vi "AuMT8852B EDR Rel Outp Pwr Extended Test.vi"() -> ()   [LabVIEW 2017]
doc: "This example shows how to extract Extended Test Results by using multiple 'Results Panels', each configurable via the 'Stage' Configuration Input control. Note that the 'Configuration Settings' (i.e. Use Low/Medium/High Frequency), must be enabled in order to obtain valid test results in the appropriate 'Test Results' output panel."
panel:
  out "error out":errorcluster
  in  "Settings":T1={"Low frequency selection"=enum."Use low frequency", "Medium frequency selection"=enum."Use medium frequency", "High frequency selection"=enum."Use high frequency", "Low TX frequency"=2402.0, "Low RX frequency"=2480.0, "Medium TX frequency"=2441.0, "Medium RX frequency"=2402.0, "High TX frequency"=2480.0, "High RX frequency"=2402.0, "Number of packets"=10, "PDPSK-PGFSK upper limit (dB) "=1.0, "PDPSK-PGFSK lower limit (dB)"=4.0, "2DHx test packet"=enum."Longest", "3DHx test packet"=enum."Longest", "Hop selection"=enum."Test with hopping off and on", "Test control"=enum."Loopback", "Hop mode"=enum."Defined", "Output Power Level"=enum."Max & Min"} {"PDPSK-PGFSK lower limit (dB)" format="%.2f"; "PDPSK-PGFSK upper limit (dB)" format="%.2f"}
  out "Addresses":string[](array[string])
  in  "Start/Stop (Start)":enum16{"Start", "Stop"}(ring)
  in  "Test Results":T2(tab)=enum."Hopon any Max"
  in  "Stage 1":T3(ring)
  out "Results 1":T4 {"Peak 2DHx DPSK Absolute Power (dBm)" format="%.2f"; "Avg 2DHx DPSK Absolute Power (dBm)" format="%.2f"; "Min 2DHx DPSK Absolute Power (dBm)" format="%.2f"; "Max 2DHx DPSK Absolute Power (dBm)" format="%.2f"; "Peak 2DHx GFSK Absolute Power (dBm)" format="%.2f"; "Avg 2DHx GFSK Absolute Power (dBm)" format="%.2f"; "Min 2DHx GFSK Absolute Power (dBm)" format="%.2f"; "Max 2DHx GFSK Absolute Power (dBm)" format="%.2f"; "Peak 3DHx DPSK Absolute Power (dBm)" format="%.2f"; "Avg 3DHx DPSK Absolute Power (dBm)" format="%.2f"; "Min 3DHx DPSK Absolute Power (dBm)" format="%.2f"; "Max 3DHx DPSK Absolute Power (dBm)" format="%.2f"; "Peak 3DHx GFSK Absolute Power (dBm)" format="%.2f"; "Avg 3DHx GFSK Absolute Power (dBm)" format="%.2f"; "Min 3DHx GFSK Absolute Power (dBm)" format="%.2f"; "Max 3DHx GFSK Absolute Power (dBm)" format="%.2f"; "Avg power difference (dBm)" format="%.2f"; "Min power difference (dBm)" format="%.2f"; "Max power difference (dBm)" format="%.2f"; "Avg power difference (dBm)" format="%.2f"; "Min power difference (dBm)" format="%.2f"; "Max power difference (dBm)" format="%.2f"}
  in  "Stage 2":T3(ring)=enum."Hop off defined low frequency EUT Max"
  out "Results  2":T4 {"Peak 2DHx DPSK Absolute Power (dBm)" format="%.2f"; "Avg 2DHx DPSK Absolute Power (dBm)" format="%.2f"; "Min 2DHx DPSK Absolute Power (dBm)" format="%.2f"; "Max 2DHx DPSK Absolute Power (dBm)" format="%.2f"; "Peak 2DHx GFSK Absolute Power (dBm)" format="%.2f"; "Avg 2DHx GFSK Absolute Power (dBm)" format="%.2f"; "Min 2DHx GFSK Absolute Power (dBm)" format="%.2f"; "Max 2DHx GFSK Absolute Power (dBm)" format="%.2f"; "Peak 3DHx DPSK Absolute Power (dBm)" format="%.2f"; "Avg 3DHx DPSK Absolute Power (dBm)" format="%.2f"; "Min 3DHx DPSK Absolute Power (dBm)" format="%.2f"; "Max 3DHx DPSK Absolute Power (dBm)" format="%.2f"; "Peak 3DHx GFSK Absolute Power (dBm)" format="%.2f"; "Avg 3DHx GFSK Absolute Power (dBm)" format="%.2f"; "Min 3DHx GFSK Absolute Power (dBm)" format="%.2f"; "Max 3DHx GFSK Absolute Power (dBm)" format="%.2f"; "Avg power difference (dBm)" format="%.2f"; "Min power difference (dBm)" format="%.2f"; "Max power difference (dBm)" format="%.2f"; "Avg power difference (dBm)" format="%.2f"; "Min power difference (dBm)" format="%.2f"; "Max power difference (dBm)" format="%.2f"}
  in  "Stage 3":T3(ring)=enum."Hop off defined medium frequency EUT Min"
  out "Results  3":T4 {"Peak 2DHx DPSK Absolute Power (dBm)" format="%.2f"; "Avg 2DHx DPSK Absolute Power (dBm)" format="%.2f"; "Min 2DHx DPSK Absolute Power (dBm)" format="%.2f"; "Max 2DHx DPSK Absolute Power (dBm)" format="%.2f"; "Peak 2DHx GFSK Absolute Power (dBm)" format="%.2f"; "Avg 2DHx GFSK Absolute Power (dBm)" format="%.2f"; "Min 2DHx GFSK Absolute Power (dBm)" format="%.2f"; "Max 2DHx GFSK Absolute Power (dBm)" format="%.2f"; "Peak 3DHx DPSK Absolute Power (dBm)" format="%.2f"; "Avg 3DHx DPSK Absolute Power (dBm)" format="%.2f"; "Min 3DHx DPSK Absolute Power (dBm)" format="%.2f"; "Max 3DHx DPSK Absolute Power (dBm)" format="%.2f"; "Peak 3DHx GFSK Absolute Power (dBm)" format="%.2f"; "Avg 3DHx GFSK Absolute Power (dBm)" format="%.2f"; "Min 3DHx GFSK Absolute Power (dBm)" format="%.2f"; "Max 3DHx GFSK Absolute Power (dBm)" format="%.2f"; "Avg power difference (dBm)" format="%.2f"; "Min power difference (dBm)" format="%.2f"; "Max power difference (dBm)" format="%.2f"; "Avg power difference (dBm)" format="%.2f"; "Min power difference (dBm)" format="%.2f"; "Max power difference (dBm)" format="%.2f"}
  in  "Stage 4":T3(ring)=enum."Hop off defined medium frequency EUT Max"
  out "Results  4":T4 {"Peak 2DHx DPSK Absolute Power (dBm)" format="%.2f"; "Avg 2DHx DPSK Absolute Power (dBm)" format="%.2f"; "Min 2DHx DPSK Absolute Power (dBm)" format="%.2f"; "Max 2DHx DPSK Absolute Power (dBm)" format="%.2f"; "Peak 2DHx GFSK Absolute Power (dBm)" format="%.2f"; "Avg 2DHx GFSK Absolute Power (dBm)" format="%.2f"; "Min 2DHx GFSK Absolute Power (dBm)" format="%.2f"; "Max 2DHx GFSK Absolute Power (dBm)" format="%.2f"; "Peak 3DHx DPSK Absolute Power (dBm)" format="%.2f"; "Avg 3DHx DPSK Absolute Power (dBm)" format="%.2f"; "Min 3DHx DPSK Absolute Power (dBm)" format="%.2f"; "Max 3DHx DPSK Absolute Power (dBm)" format="%.2f"; "Peak 3DHx GFSK Absolute Power (dBm)" format="%.2f"; "Avg 3DHx GFSK Absolute Power (dBm)" format="%.2f"; "Min 3DHx GFSK Absolute Power (dBm)" format="%.2f"; "Max 3DHx GFSK Absolute Power (dBm)" format="%.2f"; "Avg power difference (dBm)" format="%.2f"; "Min power difference (dBm)" format="%.2f"; "Max power difference (dBm)" format="%.2f"; "Avg power difference (dBm)" format="%.2f"; "Min power difference (dBm)" format="%.2f"; "Max power difference (dBm)" format="%.2f"}
  in  "Stage 5":T3(ring)=enum."Hop off defined high frequency EUT Min"
  out "Results  5":T4 {"Peak 2DHx DPSK Absolute Power (dBm)" format="%.2f"; "Avg 2DHx DPSK Absolute Power (dBm)" format="%.2f"; "Min 2DHx DPSK Absolute Power (dBm)" format="%.2f"; "Max 2DHx DPSK Absolute Power (dBm)" format="%.2f"; "Peak 2DHx GFSK Absolute Power (dBm)" format="%.2f"; "Avg 2DHx GFSK Absolute Power (dBm)" format="%.2f"; "Min 2DHx GFSK Absolute Power (dBm)" format="%.2f"; "Max 2DHx GFSK Absolute Power (dBm)" format="%.2f"; "Peak 3DHx DPSK Absolute Power (dBm)" format="%.2f"; "Avg 3DHx DPSK Absolute Power (dBm)" format="%.2f"; "Min 3DHx DPSK Absolute Power (dBm)" format="%.2f"; "Max 3DHx DPSK Absolute Power (dBm)" format="%.2f"; "Peak 3DHx GFSK Absolute Power (dBm)" format="%.2f"; "Avg 3DHx GFSK Absolute Power (dBm)" format="%.2f"; "Min 3DHx GFSK Absolute Power (dBm)" format="%.2f"; "Max 3DHx GFSK Absolute Power (dBm)" format="%.2f"; "Avg power difference (dBm)" format="%.2f"; "Min power difference (dBm)" format="%.2f"; "Max power difference (dBm)" format="%.2f"; "Avg power difference (dBm)" format="%.2f"; "Min power difference (dBm)" format="%.2f"; "Max power difference (dBm)" format="%.2f"}
  in  "Stage 6":T3(ring)=enum."Hop off defined high frequency EUT Max"
  out "Results  6":T4 {"Peak 2DHx DPSK Absolute Power (dBm)" format="%.2f"; "Avg 2DHx DPSK Absolute Power (dBm)" format="%.2f"; "Min 2DHx DPSK Absolute Power (dBm)" format="%.2f"; "Max 2DHx DPSK Absolute Power (dBm)" format="%.2f"; "Peak 2DHx GFSK Absolute Power (dBm)" format="%.2f"; "Avg 2DHx GFSK Absolute Power (dBm)" format="%.2f"; "Min 2DHx GFSK Absolute Power (dBm)" format="%.2f"; "Max 2DHx GFSK Absolute Power (dBm)" format="%.2f"; "Peak 3DHx DPSK Absolute Power (dBm)" format="%.2f"; "Avg 3DHx DPSK Absolute Power (dBm)" format="%.2f"; "Min 3DHx DPSK Absolute Power (dBm)" format="%.2f"; "Max 3DHx DPSK Absolute Power (dBm)" format="%.2f"; "Peak 3DHx GFSK Absolute Power (dBm)" format="%.2f"; "Avg 3DHx GFSK Absolute Power (dBm)" format="%.2f"; "Min 3DHx GFSK Absolute Power (dBm)" format="%.2f"; "Max 3DHx GFSK Absolute Power (dBm)" format="%.2f"; "Avg power difference (dBm)" format="%.2f"; "Min power difference (dBm)" format="%.2f"; "Max power difference (dBm)" format="%.2f"; "Avg power difference (dBm)" format="%.2f"; "Min power difference (dBm)" format="%.2f"; "Max power difference (dBm)" format="%.2f"}
  in  "Stage 7":T3(ring)=enum."Hop on defined low frequency EUT Min"
  out "Results  7":T4 {"Peak 2DHx DPSK Absolute Power (dBm)" format="%.2f"; "Avg 2DHx DPSK Absolute Power (dBm)" format="%.2f"; "Min 2DHx DPSK Absolute Power (dBm)" format="%.2f"; "Max 2DHx DPSK Absolute Power (dBm)" format="%.2f"; "Peak 2DHx GFSK Absolute Power (dBm)" format="%.2f"; "Avg 2DHx GFSK Absolute Power (dBm)" format="%.2f"; "Min 2DHx GFSK Absolute Power (dBm)" format="%.2f"; "Max 2DHx GFSK Absolute Power (dBm)" format="%.2f"; "Peak 3DHx DPSK Absolute Power (dBm)" format="%.2f"; "Avg 3DHx DPSK Absolute Power (dBm)" format="%.2f"; "Min 3DHx DPSK Absolute Power (dBm)" format="%.2f"; "Max 3DHx DPSK Absolute Power (dBm)" format="%.2f"; "Peak 3DHx GFSK Absolute Power (dBm)" format="%.2f"; "Avg 3DHx GFSK Absolute Power (dBm)" format="%.2f"; "Min 3DHx GFSK Absolute Power (dBm)" format="%.2f"; "Max 3DHx GFSK Absolute Power (dBm)" format="%.2f"; "Avg power difference (dBm)" format="%.2f"; "Min power difference (dBm)" format="%.2f"; "Max power difference (dBm)" format="%.2f"; "Avg power difference (dBm)" format="%.2f"; "Min power difference (dBm)" format="%.2f"; "Max power difference (dBm)" format="%.2f"}
  in  "Stage 8":T3(ring)=enum."Hop on defined low frequency EUT Max"
  out "Results  8":T4 {"Peak 2DHx DPSK Absolute Power (dBm)" format="%.2f"; "Avg 2DHx DPSK Absolute Power (dBm)" format="%.2f"; "Min 2DHx DPSK Absolute Power (dBm)" format="%.2f"; "Max 2DHx DPSK Absolute Power (dBm)" format="%.2f"; "Peak 2DHx GFSK Absolute Power (dBm)" format="%.2f"; "Avg 2DHx GFSK Absolute Power (dBm)" format="%.2f"; "Min 2DHx GFSK Absolute Power (dBm)" format="%.2f"; "Max 2DHx GFSK Absolute Power (dBm)" format="%.2f"; "Peak 3DHx DPSK Absolute Power (dBm)" format="%.2f"; "Avg 3DHx DPSK Absolute Power (dBm)" format="%.2f"; "Min 3DHx DPSK Absolute Power (dBm)" format="%.2f"; "Max 3DHx DPSK Absolute Power (dBm)" format="%.2f"; "Peak 3DHx GFSK Absolute Power (dBm)" format="%.2f"; "Avg 3DHx GFSK Absolute Power (dBm)" format="%.2f"; "Min 3DHx GFSK Absolute Power (dBm)" format="%.2f"; "Max 3DHx GFSK Absolute Power (dBm)" format="%.2f"; "Avg power difference (dBm)" format="%.2f"; "Min power difference (dBm)" format="%.2f"; "Max power difference (dBm)" format="%.2f"; "Avg power difference (dBm)" format="%.2f"; "Min power difference (dBm)" format="%.2f"; "Max power difference (dBm)" format="%.2f"}
  in  "Stage 9":T3(ring)=enum."Hop on defined medium frequency EUT Min"
  out "Results  9":T4 {"Peak 2DHx DPSK Absolute Power (dBm)" format="%.2f"; "Avg 2DHx DPSK Absolute Power (dBm)" format="%.2f"; "Min 2DHx DPSK Absolute Power (dBm)" format="%.2f"; "Max 2DHx DPSK Absolute Power (dBm)" format="%.2f"; "Peak 2DHx GFSK Absolute Power (dBm)" format="%.2f"; "Avg 2DHx GFSK Absolute Power (dBm)" format="%.2f"; "Min 2DHx GFSK Absolute Power (dBm)" format="%.2f"; "Max 2DHx GFSK Absolute Power (dBm)" format="%.2f"; "Peak 3DHx DPSK Absolute Power (dBm)" format="%.2f"; "Avg 3DHx DPSK Absolute Power (dBm)" format="%.2f"; "Min 3DHx DPSK Absolute Power (dBm)" format="%.2f"; "Max 3DHx DPSK Absolute Power (dBm)" format="%.2f"; "Peak 3DHx GFSK Absolute Power (dBm)" format="%.2f"; "Avg 3DHx GFSK Absolute Power (dBm)" format="%.2f"; "Min 3DHx GFSK Absolute Power (dBm)" format="%.2f"; "Max 3DHx GFSK Absolute Power (dBm)" format="%.2f"; "Avg power difference (dBm)" format="%.2f"; "Min power difference (dBm)" format="%.2f"; "Max power difference (dBm)" format="%.2f"; "Avg power difference (dBm)" format="%.2f"; "Min power difference (dBm)" format="%.2f"; "Max power difference (dBm)" format="%.2f"}
  in  "Stage 10":T3(ring)=enum."Hop on defined medium frequency EUT Max"
  out "Results  10":T4 {"Peak 2DHx DPSK Absolute Power (dBm)" format="%.2f"; "Avg 2DHx DPSK Absolute Power (dBm)" format="%.2f"; "Min 2DHx DPSK Absolute Power (dBm)" format="%.2f"; "Max 2DHx DPSK Absolute Power (dBm)" format="%.2f"; "Peak 2DHx GFSK Absolute Power (dBm)" format="%.2f"; "Avg 2DHx GFSK Absolute Power (dBm)" format="%.2f"; "Min 2DHx GFSK Absolute Power (dBm)" format="%.2f"; "Max 2DHx GFSK Absolute Power (dBm)" format="%.2f"; "Peak 3DHx DPSK Absolute Power (dBm)" format="%.2f"; "Avg 3DHx DPSK Absolute Power (dBm)" format="%.2f"; "Min 3DHx DPSK Absolute Power (dBm)" format="%.2f"; "Max 3DHx DPSK Absolute Power (dBm)" format="%.2f"; "Peak 3DHx GFSK Absolute Power (dBm)" format="%.2f"; "Avg 3DHx GFSK Absolute Power (dBm)" format="%.2f"; "Min 3DHx GFSK Absolute Power (dBm)" format="%.2f"; "Max 3DHx GFSK Absolute Power (dBm)" format="%.2f"; "Avg power difference (dBm)" format="%.2f"; "Min power difference (dBm)" format="%.2f"; "Max power difference (dBm)" format="%.2f"; "Avg power difference (dBm)" format="%.2f"; "Min power difference (dBm)" format="%.2f"; "Max power difference (dBm)" format="%.2f"}
  in  "Stage 11":T3(ring)=enum."Hop on defined high frequency EUT Min"
  out "Results  11":T4 {"Peak 2DHx DPSK Absolute Power (dBm)" format="%.2f"; "Avg 2DHx DPSK Absolute Power (dBm)" format="%.2f"; "Min 2DHx DPSK Absolute Power (dBm)" format="%.2f"; "Max 2DHx DPSK Absolute Power (dBm)" format="%.2f"; "Peak 2DHx GFSK Absolute Power (dBm)" format="%.2f"; "Avg 2DHx GFSK Absolute Power (dBm)" format="%.2f"; "Min 2DHx GFSK Absolute Power (dBm)" format="%.2f"; "Max 2DHx GFSK Absolute Power (dBm)" format="%.2f"; "Peak 3DHx DPSK Absolute Power (dBm)" format="%.2f"; "Avg 3DHx DPSK Absolute Power (dBm)" format="%.2f"; "Min 3DHx DPSK Absolute Power (dBm)" format="%.2f"; "Max 3DHx DPSK Absolute Power (dBm)" format="%.2f"; "Peak 3DHx GFSK Absolute Power (dBm)" format="%.2f"; "Avg 3DHx GFSK Absolute Power (dBm)" format="%.2f"; "Min 3DHx GFSK Absolute Power (dBm)" format="%.2f"; "Max 3DHx GFSK Absolute Power (dBm)" format="%.2f"; "Avg power difference (dBm)" format="%.2f"; "Min power difference (dBm)" format="%.2f"; "Max power difference (dBm)" format="%.2f"; "Avg power difference (dBm)" format="%.2f"; "Min power difference (dBm)" format="%.2f"; "Max power difference (dBm)" format="%.2f"}
  in  "Stage 12":T3(ring)=enum."Hop on defined high frequency EUT Max"
  out "Results  12":T4 {"Peak 2DHx DPSK Absolute Power (dBm)" format="%.2f"; "Avg 2DHx DPSK Absolute Power (dBm)" format="%.2f"; "Min 2DHx DPSK Absolute Power (dBm)" format="%.2f"; "Max 2DHx DPSK Absolute Power (dBm)" format="%.2f"; "Peak 2DHx GFSK Absolute Power (dBm)" format="%.2f"; "Avg 2DHx GFSK Absolute Power (dBm)" format="%.2f"; "Min 2DHx GFSK Absolute Power (dBm)" format="%.2f"; "Max 2DHx GFSK Absolute Power (dBm)" format="%.2f"; "Peak 3DHx DPSK Absolute Power (dBm)" format="%.2f"; "Avg 3DHx DPSK Absolute Power (dBm)" format="%.2f"; "Min 3DHx DPSK Absolute Power (dBm)" format="%.2f"; "Max 3DHx DPSK Absolute Power (dBm)" format="%.2f"; "Peak 3DHx GFSK Absolute Power (dBm)" format="%.2f"; "Avg 3DHx GFSK Absolute Power (dBm)" format="%.2f"; "Min 3DHx GFSK Absolute Power (dBm)" format="%.2f"; "Max 3DHx GFSK Absolute Power (dBm)" format="%.2f"; "Avg power difference (dBm)" format="%.2f"; "Min power difference (dBm)" format="%.2f"; "Max power difference (dBm)" format="%.2f"; "Avg power difference (dBm)" format="%.2f"; "Min power difference (dBm)" format="%.2f"; "Max power difference (dBm)" format="%.2f"}
  in  "Stage 13":T3(ring)=enum."Hop on all channels EUT Min"
  out "Results  13":T4 {"Peak 2DHx DPSK Absolute Power (dBm)" format="%.2f"; "Avg 2DHx DPSK Absolute Power (dBm)" format="%.2f"; "Min 2DHx DPSK Absolute Power (dBm)" format="%.2f"; "Max 2DHx DPSK Absolute Power (dBm)" format="%.2f"; "Peak 2DHx GFSK Absolute Power (dBm)" format="%.2f"; "Avg 2DHx GFSK Absolute Power (dBm)" format="%.2f"; "Min 2DHx GFSK Absolute Power (dBm)" format="%.2f"; "Max 2DHx GFSK Absolute Power (dBm)" format="%.2f"; "Peak 3DHx DPSK Absolute Power (dBm)" format="%.2f"; "Avg 3DHx DPSK Absolute Power (dBm)" format="%.2f"; "Min 3DHx DPSK Absolute Power (dBm)" format="%.2f"; "Max 3DHx DPSK Absolute Power (dBm)" format="%.2f"; "Peak 3DHx GFSK Absolute Power (dBm)" format="%.2f"; "Avg 3DHx GFSK Absolute Power (dBm)" format="%.2f"; "Min 3DHx GFSK Absolute Power (dBm)" format="%.2f"; "Max 3DHx GFSK Absolute Power (dBm)" format="%.2f"; "Avg power difference (dBm)" format="%.2f"; "Min power difference (dBm)" format="%.2f"; "Max power difference (dBm)" format="%.2f"; "Avg power difference (dBm)" format="%.2f"; "Min power difference (dBm)" format="%.2f"; "Max power difference (dBm)" format="%.2f"}
  in  "Stage 14":T3(ring)=enum."Hop on all channels EUT Max"
  out "Results  14":T4 {"Peak 2DHx DPSK Absolute Power (dBm)" format="%.2f"; "Avg 2DHx DPSK Absolute Power (dBm)" format="%.2f"; "Min 2DHx DPSK Absolute Power (dBm)" format="%.2f"; "Max 2DHx DPSK Absolute Power (dBm)" format="%.2f"; "Peak 2DHx GFSK Absolute Power (dBm)" format="%.2f"; "Avg 2DHx GFSK Absolute Power (dBm)" format="%.2f"; "Min 2DHx GFSK Absolute Power (dBm)" format="%.2f"; "Max 2DHx GFSK Absolute Power (dBm)" format="%.2f"; "Peak 3DHx DPSK Absolute Power (dBm)" format="%.2f"; "Avg 3DHx DPSK Absolute Power (dBm)" format="%.2f"; "Min 3DHx DPSK Absolute Power (dBm)" format="%.2f"; "Max 3DHx DPSK Absolute Power (dBm)" format="%.2f"; "Peak 3DHx GFSK Absolute Power (dBm)" format="%.2f"; "Avg 3DHx GFSK Absolute Power (dBm)" format="%.2f"; "Min 3DHx GFSK Absolute Power (dBm)" format="%.2f"; "Max 3DHx GFSK Absolute Power (dBm)" format="%.2f"; "Avg power difference (dBm)" format="%.2f"; "Min power difference (dBm)" format="%.2f"; "Max power difference (dBm)" format="%.2f"; "Avg power difference (dBm)" format="%.2f"; "Min power difference (dBm)" format="%.2f"; "Max power difference (dBm)" format="%.2f"}
  in  "Stage 15":T3(ring)=enum."Hop on any channels EUT Min"
  out "Results  15":T4 {"Peak 2DHx DPSK Absolute Power (dBm)" format="%.2f"; "Avg 2DHx DPSK Absolute Power (dBm)" format="%.2f"; "Min 2DHx DPSK Absolute Power (dBm)" format="%.2f"; "Max 2DHx DPSK Absolute Power (dBm)" format="%.2f"; "Peak 2DHx GFSK Absolute Power (dBm)" format="%.2f"; "Avg 2DHx GFSK Absolute Power (dBm)" format="%.2f"; "Min 2DHx GFSK Absolute Power (dBm)" format="%.2f"; "Max 2DHx GFSK Absolute Power (dBm)" format="%.2f"; "Peak 3DHx DPSK Absolute Power (dBm)" format="%.2f"; "Avg 3DHx DPSK Absolute Power (dBm)" format="%.2f"; "Min 3DHx DPSK Absolute Power (dBm)" format="%.2f"; "Max 3DHx DPSK Absolute Power (dBm)" format="%.2f"; "Peak 3DHx GFSK Absolute Power (dBm)" format="%.2f"; "Avg 3DHx GFSK Absolute Power (dBm)" format="%.2f"; "Min 3DHx GFSK Absolute Power (dBm)" format="%.2f"; "Max 3DHx GFSK Absolute Power (dBm)" format="%.2f"; "Avg power difference (dBm)" format="%.2f"; "Min power difference (dBm)" format="%.2f"; "Max power difference (dBm)" format="%.2f"; "Avg power difference (dBm)" format="%.2f"; "Min power difference (dBm)" format="%.2f"; "Max power difference (dBm)" format="%.2f"}
  in  "Stage 16":T3(ring)=enum."Hop on any channels EUT Max"
  out "Results  16":T4 {"Peak 2DHx DPSK Absolute Power (dBm)" format="%.2f"; "Avg 2DHx DPSK Absolute Power (dBm)" format="%.2f"; "Min 2DHx DPSK Absolute Power (dBm)" format="%.2f"; "Max 2DHx DPSK Absolute Power (dBm)" format="%.2f"; "Peak 2DHx GFSK Absolute Power (dBm)" format="%.2f"; "Avg 2DHx GFSK Absolute Power (dBm)" format="%.2f"; "Min 2DHx GFSK Absolute Power (dBm)" format="%.2f"; "Max 2DHx GFSK Absolute Power (dBm)" format="%.2f"; "Peak 3DHx DPSK Absolute Power (dBm)" format="%.2f"; "Avg 3DHx DPSK Absolute Power (dBm)" format="%.2f"; "Min 3DHx DPSK Absolute Power (dBm)" format="%.2f"; "Max 3DHx DPSK Absolute Power (dBm)" format="%.2f"; "Peak 3DHx GFSK Absolute Power (dBm)" format="%.2f"; "Avg 3DHx GFSK Absolute Power (dBm)" format="%.2f"; "Min 3DHx GFSK Absolute Power (dBm)" format="%.2f"; "Max 3DHx GFSK Absolute Power (dBm)" format="%.2f"; "Avg power difference (dBm)" format="%.2f"; "Min power difference (dBm)" format="%.2f"; "Max power difference (dBm)" format="%.2f"; "Avg power difference (dBm)" format="%.2f"; "Min power difference (dBm)" format="%.2f"; "Max power difference (dBm)" format="%.2f"}
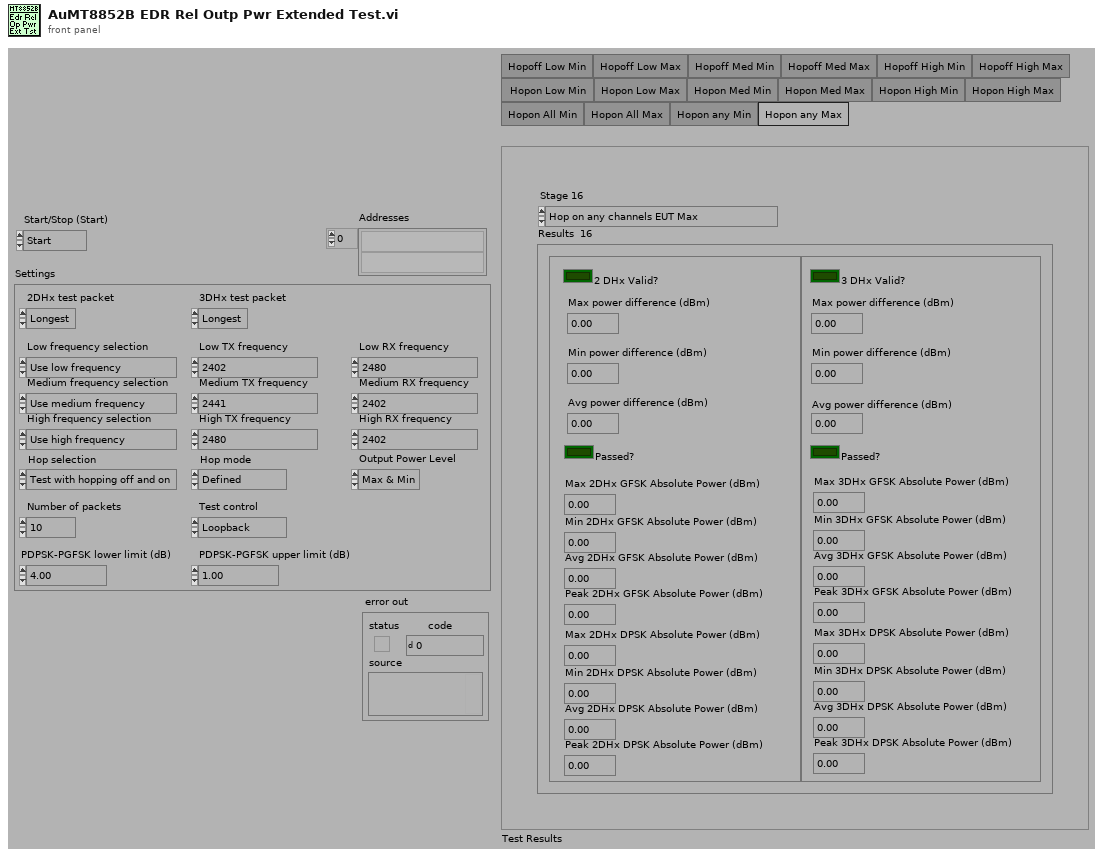
[diagram p1: front panel]
types:
  T1 = cluster{"Low frequency selection":enum16{"Don't use low frequency", "Use low frequency"}, "Medium frequency selection":enum16{"Don't use medium frequency", "Use medium frequency"}, "High frequency selection":enum16{"Don't use high frequency", "Use high frequency"}, "Low TX frequency":dbl, "Low RX frequency":dbl, "Medium TX frequency":dbl, "Medium RX frequency":dbl, "High TX frequency":dbl, "High RX frequency":dbl, "Number of packets":i32, "PDPSK-PGFSK upper limit (dB) ":dbl, "PDPSK-PGFSK lower limit (dB)":dbl, "2DHx test packet":enum16{"OFF", "Longest", "2-DH1", "2-DH3", "2-DH5"}, "3DHx test packet":enum16{"OFF", "Longest", "3-DH1", "3-DH3", "3-DH5"}, "Hop selection":enum16{"Test with hopping on", "Test with hopping off", "Test with hopping off and on"}, "Test control":enum16{"Loopback", "TX test"}, "Hop mode":enum16{"All", "Any", "Defined"}, "Output Power Level":enum16{"Min only", "Max only", "Max & Min"}}
  T2 = enum32{"Hopoff Low Min", "Hopoff Low Max", "Hopoff Med Min", "Hopoff Med Max", "Hopoff High Min", "Hopoff High Max", "Hopon Low Min ", "Hopon Low Max", "Hopon Med Min", "Hopon Med Max", "Hopon High Min", "Hopon High Max", "Hopon All Min", "Hopon All Max", "Hopon any Min", "Hopon any Max"}
  T3 = enum16{"Hop off defined low frequency EUT Min", "Hop off defined low frequency EUT Max", "Hop off defined medium frequency EUT Min", "Hop off defined medium frequency EUT Max", "Hop off defined high frequency EUT Min", "Hop off defined high frequency EUT Max", "Hop on defined low frequency EUT Min", "Hop on defined low frequency EUT Max", "Hop on defined medium frequency EUT Min", "Hop on defined medium frequency EUT Max", "Hop on defined high frequency EUT Min", "Hop on defined high frequency EUT Max", "Hop on all channels EUT Min", "Hop on all channels EUT Max", "Hop on any channels EUT Min", "Hop on any channels EUT Max"}
  T4 = cluster{"2 DHx Valid?":bool, "Max power difference (dBm)":dbl, "Min power difference (dBm)":dbl, "Avg power difference (dBm)":dbl, "Passed?":bool, "3 DHx Valid?":bool, "Max power difference (dBm)":dbl, "Min power difference (dBm)":dbl, "Avg power difference (dBm)":dbl, "Passed?":bool, "Max 3DHx GFSK Absolute Power (dBm)":dbl, "Min 3DHx GFSK Absolute Power (dBm)":dbl, "Avg 3DHx GFSK Absolute Power (dBm)":dbl, "Peak 3DHx GFSK Absolute Power (dBm)":dbl, "Max 3DHx DPSK Absolute Power (dBm)":dbl, "Min 3DHx DPSK Absolute Power (dBm)":dbl, "Avg 3DHx DPSK Absolute Power (dBm)":dbl, "Peak 3DHx DPSK Absolute Power (dBm)":dbl, "Max 2DHx GFSK Absolute Power (dBm)":dbl, "Min 2DHx GFSK Absolute Power (dBm)":dbl, "Avg 2DHx GFSK Absolute Power (dBm)":dbl, "Peak 2DHx GFSK Absolute Power (dBm)":dbl, "Max 2DHx DPSK Absolute Power (dBm)":dbl, "Min 2DHx DPSK Absolute Power (dBm)":dbl, "Avg 2DHx DPSK Absolute Power (dBm)":dbl, "Peak 2DHx DPSK Absolute Power (dBm)":dbl}
  T5 = cluster{"Event status":enum16{"Event status disabled", "Event status enabled"}, "Message":enum16{"Message available disabled", "Message available enabled"}, "EUT Power State":u16, "State change":enum16{"State change disabled", "State change enabled"}, "Test failure":enum16{"Test failure disabled", "Test failure enabled"}, "Instrument status":enum16{"Instrument status disabled", "Instrument status enabled"}}
  T6 = cluster{"Completion":enum16{"Completion event disabled", "Completion event enabled"}, "Disconnect":enum16{"Disconnect event disabled", "Disconnect event enabled"}, "Connect":enum16{"Connect event disabled", "Connect event enabled"}, "Inquiry":enum16{"Inquiry event disabled", "Inquiry event enabled"}, "Temperature":enum16{"Temperature warning disabled", "Temperature warning enabled"}}
  T7 = cluster{"Reset":enum16{"Don't reset", "Reset"}, "Identity checking":enum16{"Don't query identity", "Query identity"}, "Simulation":enum16{"Don't simulate", "Simulate"}, "Range checking":enum16{"Don't check attribute ranges", "Check attribute ranges"}, "State caching":enum16{"Don't cache attributes", "Cache attributes"}, "Status checking":enum16{"Don't query instrument status", "Query instrument status"}}
  T8 = cluster{"Output power (Selected)":enum16{"Output power not selected", "Output power selected"}, "Power control (Selected)":enum16{"Power control not selected", "Power control selected"}, "Modulation index (Selected)":enum16{"Modulation index not selected", "Modulation index selected"}, "Initial carrier (Selected)":enum16{"Initial carrier not selected", "Initial carrier selected"}, "Carrier drift (Selected)":enum16{"Carrier drift not selected", "Carrier drift selected"}, "Single-slot sensitivity (Selected)":enum16{"Single-slot sensitivity not selected", "Single-slot sensitivity selected"}, "Multi-slot sensitivity (Selected)":enum16{"Multi-slot sensitivity not selected", "Multi-slot sensitivity selected"}, "Maximum input power (Selected)":enum16{"Maximum input power not selected", "Maximum input power selected"}, "Relative transmit power (Selected)":enum16{"Rel. transmit power not selected", "Rel. transmit power selected"}, "Carrier frequency stability and modulation (Selected)":enum16{"Carrier freq. and stability not selected", "Carrier freq. and stability selected"}, "Differential phase encoding":enum16{"Differential phase not selected", "Differential phase selected"}, "Sensitivity (Selected)":enum16{"Sensitivity not selected", "Sensitivity selected"}, "BER floor sensitivity (Selected)":enum16{"BER floor sensitivity not selected", "BER floor sensitivity selected"}, "EDR Maximum input power (Selected)":enum16{"EDR Max input power not selected", "EDR Max input power selected"}}
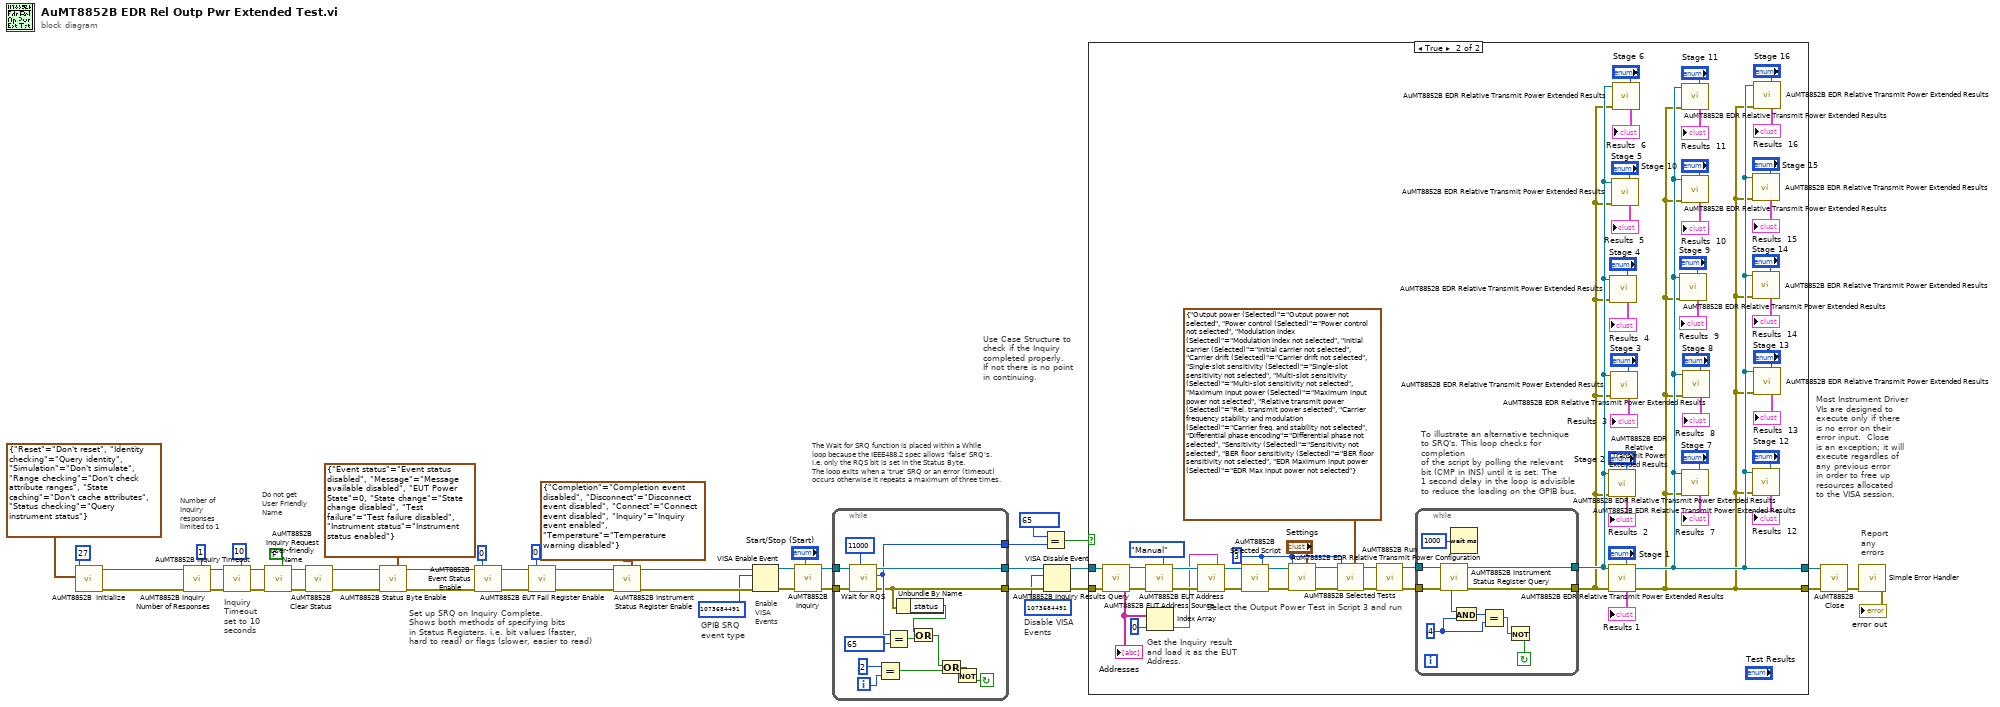
[diagram p0: block diagram]
diagram:
  # "Most Instrument Driver\nVIs are designed to\nexecute only if there \nis no error on their\nerror input.  Close \nis an exception; it will \nexecute regardles of \nany previous error\nin order to free up \nresources allocated\nto the VISA session."
  # "Report\nany \nerrors"
  # "Use Case Structure to\ncheck if the Inquiry\ncompleted properly. \nIf not there is no point \nin continuing."
  # "Disable VISA\nEvents"
  # "The Wait for SRQ function is placed within a While\nloop because the IEEE488.2 spec allows 'false' SRQ's.\ni.e. only the RQS bit is set in the Status Byte.\nThe loop exits when a 'true' SRQ or an error (timeout) \noccurs otherwise it repeats a maximum of three times."
  # "Enable\nVISA\nEvents"
  # "Set up SRQ on Inquiry Complete.\nShows both methods of specifying bits\nin Status Registers. i.e. bit values (faster, \nhard to read) or flags (slower, easier to read)"
  # "Inquiry Timeout\nset to 10 seconds"
  # "Number of\nInquiry responses\nlimited to 1"
  # "GPIB SRQ\nevent type"
  # "Do not get \nUser Friendly Name"
  n1 = call <instrlib>:"AuMT8852B  Initialize.vi"("Options"=T7 {"Reset"=enum."Don't reset", "Identity checking"=enum."Query identity", "Simulation"=enum."Don't simulate", "Range checking"=enum."Don't check attribute ranges", "State caching"=enum."Don't cache attributes", "Status checking"=enum."Query instrument status"}, "GPIB Address (27)"=27) -> ("error out"=w43:errorcluster, "VISA session out"=w44:refnum<visa-resource-name>)  [unwired: 8 in]
  n2 = call <instrlib>:"AuMT8852B Inquiry Number of Responses.vi"("Responses (1)"=1, "error in (no error)"=w43, "VISA session"=w44) -> ("error out"=w41:errorcluster, "VISA session out"=w42:refnum<visa-resource-name>)  [unwired: 5 in, 2 out]
  n3 = call <instrlib>:"AuMT8852B Inquiry Timeout.vi"("Timeout (1)"=10, "error in (no error)"=w41, "VISA session"=w42) -> ("error out"=w38:errorcluster, "VISA session out"=w39:refnum<visa-resource-name>)  [unwired: 5 in, 2 out]
  n4 = call <instrlib>:"AuMT8852B Inquiry Request User-friendly Name.vi"("Status (T)"=FALSE, "error in (no error)"=w38, "VISA session"=w39) -> ("error out"=w33:errorcluster, "VISA session out"=w34:refnum<visa-resource-name>)  [unwired: 5 in, 2 out]
  n5 = call <instrlib>:"AuMT8852B Clear Status.vi"("error in (no error)"=w33, "VISA session"=w34) -> ("error out"=w31:errorcluster, "VISA session out"=w32:refnum<visa-resource-name>)  [unwired: 7 in, 1 out]
  n6 = call <instrlib>:"AuMT8852B Status Byte Enable.vi"("Flags in (all disabled)"=T5 {"Event status"=enum."Event status disabled", "Message"=enum."Message available disabled", "EUT Power State"=0, "State change"=enum."State change disabled", "Test failure"=enum."Test failure disabled", "Instrument status"=enum."Instrument status enabled"}, "error in (no error)"=w31, "VISA session"=w32) -> ("error out"=w30:errorcluster, "VISA session out"=w27:refnum<visa-resource-name>)  [unwired: 4 in, 3 out]
  n7 = call <instrlib>:"AuMT8852B Event Status Enable.vi"("error in (no error)"=w30, "Value (-1)"=0, "VISA session"=w27) -> ("error out"=w29:errorcluster, "VISA session out"=w26:refnum<visa-resource-name>)  [unwired: 4 in, 3 out]
  n8 = call <instrlib>:"AuMT8852B EUT Fail Register Enable.vi"("error in (no error)"=w29, "Value (-1)"=0, "VISA session"=w26) -> ("error out"=w28:errorcluster, "VISA session out"=w25:refnum<visa-resource-name>)  [unwired: 4 in, 3 out]
  n9 = call <instrlib>:"AuMT8852B Instrument Status Register Enable.vi"("Flags"=T6 {"Completion"=enum."Completion event disabled", "Disconnect"=enum."Disconnect event disabled", "Connect"=enum."Connect event disabled", "Inquiry"=enum."Inquiry event enabled", "Temperature"=enum."Temperature warning disabled"}, "error in (no error)"=w28, "VISA session"=w25) -> ("error out"=w20:errorcluster, "VISA session out"=w21:refnum<visa-resource-name>)  [unwired: 4 in, 3 out]
  n10 = VISA Enable Event(8:w20, 10:u32 1073684491 ("event type"), 11:w21) -> (0:w18:errorcluster, 3:w19:refnum<visa-resource-name>)  [unwired: 1 in]
  n11 = call <instrlib>:"AuMT8852B Inquiry.vi"("Start/Stop (Start)"="Start/Stop (Start)", "error in (no error)"=w18, "VISA session"=w19) -> ("error out"=w16:errorcluster, "VISA session out"=w17:refnum<visa-resource-name>)  [unwired: 6 in, 1 out]
  n12 = while {
    tunnel: w17 -> [w60]
    tunnel: w16 -> [w59]
    tunnel: [w58] -> w15
    tunnel: [w50] -> w14
    tunnel: [w51] -> w8
    i -> [w55]
    stop <- w46 continue-if-true
    n13 = call <vilib>:"Wait for RQS.VI"("timeout (25000 ms)"=u32 11000 ("timeout ms"), "error in (no error)"=w59, "VISA resource name"=w60) -> ("error out"=w50:errorcluster, "status byte"=w51:u16, "VISA resource name out"=w58:refnum<visa-resource-name>)  [unwired: 6 in]
    n14 = Equal?(x=2, y=w55) -> (x = y?=w56:bool)
    n15 = Equal?(x=w51, y=u16 65) -> (x = y?=w49:bool)
    n16 = Unbundle By Name(w50) -> ("status"=w48:bool)
    n17 = Or(x=w48, y=w49) -> (x .or. y?=w47:bool)
    n18 = Or(x=w47, y=w56) -> (x .or. y?=w57:bool)
    n19 = Not(x=w57) -> (.not. x?=w46:bool)
  }
  n20 = Equal?(x=u16 65, y=w8) -> (x = y?=w9:bool)
  n21 = VISA Disable Event(8:w14, 10:u32 1073684491 ("event type"), 11:w15) -> (0:w12:errorcluster, 3:w13:refnum<visa-resource-name>)  [unwired: 1 in]
  n22 = case shown="True" w9 {
    tunnel: [w62 w65] -> w40
    tunnel: w13 -> [w62 w121]
    tunnel: w12 -> [w61 w120]
    tunnel: [w61 w63] -> w4
    frame False {
    }
    frame True {
      w100 = 3 ("Script (3)")
      # "To illustrate an alternative technique\nto SRQ's. This loop checks for completion \nof the script by polling the relevant \nbit (CMP in INS) until it is set. The \n1 second delay in the loop is advisible\nto reduce the loading on the GPIB bus."
      # "Select the Output Power Test in Script 3 and run"
      # "Get the Inquiry result\nand load it as the EUT\nAddress."
      n23 = call <instrlib>:"AuMT8852B Inquiry Results Query.vi"("error in (no error)"=w120, "VISA session"=w121) -> ("error out"=w118:errorcluster, "VISA session out"=w119:refnum<visa-resource-name>, "Addresses"=w114:string[])  [unwired: 5 in, 2 out]
      "Addresses" <- w114
      n24 = call <instrlib>:"AuMT8852B EUT Address Source.vi"("Source (Manual)"=enum16{"Manual", "RS-232", "USB", "Inquiry"}."Manual", "error in (no error)"=w118, "VISA session"=w119) -> ("error out"=w116:errorcluster, "VISA session out"=w115:refnum<visa-resource-name>)  [unwired: 5 in, 2 out]
      n25 = Index Array(array=w114, index=0 ("Index")) -> (element=w112:string)
      n26 = call <instrlib>:"AuMT8852B EUT Address.vi"("EUT Address (0x000000000000)"=w112, "error in (no error)"=w116, "VISA session"=w115) -> ("error out"=w109:errorcluster, "VISA session out"=w111:refnum<visa-resource-name>)  [unwired: 5 in, 2 out]
      n27 = call <instrlib>:"AuMT8852B Selected Script.vi"("Script (3)"=w100, "error in (no error)"=w109, "VISA session"=w111) -> ("error out"=w104:errorcluster, "VISA session out"=w102:refnum<visa-resource-name>)  [unwired: 5 in, 2 out]
      n28 = call <instrlib>:"AuMT8852B EDR Relative Transmit Power Configuration.vi"("Settings"="Settings", "error in (no error)"=w104, "Script (3)"=w100, "VISA session"=w102) -> ("error out"=w103:errorcluster, "VISA session out"=w101:refnum<visa-resource-name>)  [unwired: 4 in, 2 out]
      n29 = call <instrlib>:"AuMT8852B Selected Tests.vi"("Tests (All selected)"=T8 {"Output power (Selected)"=enum."Output power not selected", "Power control (Selected)"=enum."Power control not selected", "Modulation index (Selected)"=enum."Modulation index not selected", "Initial carrier (Selected)"=enum."Initial carrier not selected", "Carrier drift (Selected)"=enum."Carrier drift not selected", "Single-slot sensitivity (Selected)"=enum."Single-slot sensitivity not selected", "Multi-slot sensitivity (Selected)"=enum."Multi-slot sensitivity not selected", "Maximum input power (Selected)"=enum."Maximum input power not selected", "Relative transmit power (Selected)"=enum."Rel. transmit power selected", "Carrier frequency stability and modulation (Selected)"=enum."Carrier freq. and stability not selected", "Differential phase encoding"=enum."Differential phase not selected", "Sensitivity (Selected)"=enum."Sensitivity not selected", "BER floor sensitivity (Selected)"=enum."BER floor sensitivity not selected", "EDR Maximum input power (Selected)"=enum."EDR Max input power not selected"}, "error in (no error)"=w103, "Script (3)"=w100, "VISA session"=w101) -> ("error out"=w108:errorcluster, "VISA session out"=w110:refnum<visa-resource-name>)  [unwired: 4 in, 2 out]
      n30 = call <instrlib>:"AuMT8852B Run.vi"("error in (no error)"=w108, "VISA session"=w110) -> ("error out"=w106:errorcluster, "VISA session out"=w107:refnum<visa-resource-name>)  [unwired: 7 in, 1 out]
      n31 = while {
        tunnel: w107 -> [w131]
        tunnel: [w130] -> w66
        tunnel: w106 -> [w129]
        tunnel: [w128] -> w64
        stop <- w122 continue-if-true
        w123 = 4 ("y")
        n32 = call <instrlib>:"AuMT8852B Instrument Status Register Query.vi"("error in (no error)"=w129, "VISA session"=w131) -> ("error out"=w128:errorcluster, "VISA session out"=w130:refnum<visa-resource-name>, "Value"=w124:i32)  [unwired: 5 in, 2 out]
        n33 = Wait (ms)(milliseconds to wait=u32 1000) -> ()  [unwired: 1 out]
        n34 = And(x=w124, y=w123) -> (x .and. y?=w125:i32)
        n35 = Equal?(x=w125, y=w123) -> (x = y?=w126:bool)
        n36 = Not(x=w126) -> (.not. x?=w122:bool)
      }
      n37 = call <instrlib>:"AuMT8852B EDR Relative Transmit Power Extended Results.vi"("Stage"="Stage 2", "error in (no error)"=w64, "VISA session"=w66) -> ("Results"=→"Results  2":T4)  [unwired: 5 in, 3 out]
      n38 = call <instrlib>:"AuMT8852B EDR Relative Transmit Power Extended Results.vi"("Stage"="Stage 1", "error in (no error)"=w64, "VISA session"=w66) -> ("error out"=w63:errorcluster, "VISA session out"=w65:refnum<visa-resource-name>, "Results"=→"Results 1":T4)  [unwired: 5 in, 1 out]
      n39 = call <instrlib>:"AuMT8852B EDR Relative Transmit Power Extended Results.vi"("Stage"="Stage 4", "error in (no error)"=w64, "VISA session"=w66) -> ("Results"=→"Results  4":T4)  [unwired: 5 in, 3 out]
      n40 = call <instrlib>:"AuMT8852B EDR Relative Transmit Power Extended Results.vi"("Stage"="Stage 3", "error in (no error)"=w64, "VISA session"=w66) -> ("Results"=→"Results  3":T4)  [unwired: 5 in, 3 out]
      n41 = call <instrlib>:"AuMT8852B EDR Relative Transmit Power Extended Results.vi"("Stage"="Stage 5", "error in (no error)"=w64, "VISA session"=w66) -> ("Results"=→"Results  5":T4)  [unwired: 5 in, 3 out]
      n42 = call <instrlib>:"AuMT8852B EDR Relative Transmit Power Extended Results.vi"("Stage"="Stage 6", "error in (no error)"=w64, "VISA session"=w66) -> ("Results"=→"Results  6":T4)  [unwired: 5 in, 3 out]
      n43 = call <instrlib>:"AuMT8852B EDR Relative Transmit Power Extended Results.vi"("Stage"="Stage 9", "error in (no error)"=w63, "VISA session"=w65) -> ("Results"=→"Results  9":T4)  [unwired: 5 in, 3 out]
      n44 = call <instrlib>:"AuMT8852B EDR Relative Transmit Power Extended Results.vi"("Stage"="Stage 11", "error in (no error)"=w63, "VISA session"=w65) -> ("Results"=→"Results  11":T4)  [unwired: 5 in, 3 out]
      n45 = call <instrlib>:"AuMT8852B EDR Relative Transmit Power Extended Results.vi"("Stage"="Stage 10", "error in (no error)"=w63, "VISA session"=w65) -> ("Results"=→"Results  10":T4)  [unwired: 5 in, 3 out]
      n46 = call <instrlib>:"AuMT8852B EDR Relative Transmit Power Extended Results.vi"("Stage"="Stage 7", "error in (no error)"=w63, "VISA session"=w65) -> ("Results"=→"Results  7":T4)  [unwired: 5 in, 3 out]
      n47 = call <instrlib>:"AuMT8852B EDR Relative Transmit Power Extended Results.vi"("Stage"="Stage 8", "error in (no error)"=w63, "VISA session"=w65) -> ("Results"=→"Results  8":T4)  [unwired: 5 in, 3 out]
      n48 = call <instrlib>:"AuMT8852B EDR Relative Transmit Power Extended Results.vi"("Stage"="Stage 15", "error in (no error)"=w63, "VISA session"=w65) -> ("Results"=→"Results  15":T4)  [unwired: 5 in, 3 out]
      n49 = call <instrlib>:"AuMT8852B EDR Relative Transmit Power Extended Results.vi"("Stage"="Stage 14", "error in (no error)"=w63, "VISA session"=w65) -> ("Results"=→"Results  14":T4)  [unwired: 5 in, 3 out]
      n50 = call <instrlib>:"AuMT8852B EDR Relative Transmit Power Extended Results.vi"("Stage"="Stage 12", "error in (no error)"=w63, "VISA session"=w65) -> ("Results"=→"Results  12":T4)  [unwired: 5 in, 3 out]
      n51 = call <instrlib>:"AuMT8852B EDR Relative Transmit Power Extended Results.vi"("Stage"="Stage 16", "error in (no error)"=w63, "VISA session"=w65) -> ("Results"=→"Results  16":T4)  [unwired: 5 in, 3 out]
      n52 = call <instrlib>:"AuMT8852B EDR Relative Transmit Power Extended Results.vi"("Stage"="Stage 13", "error in (no error)"=w63, "VISA session"=w65) -> ("Results"=→"Results  13":T4)  [unwired: 5 in, 3 out]
    }
  }
  n53 = call <instrlib>:"AuMT8852B  Close.vi"("error in (no error)"=w4, "VISA session"=w40) -> ("error out"=w2:errorcluster)  [unwired: 8 in, 1 out]
  n54 = call <vilib>:"Simple Error Handler.vi"("error in (no error)"=w2) -> ("error out"=→"error out":errorcluster)  [unwired: 4 in, 4 out]
